vi "Executing.vi"(8 "error in (no error)":errorcluster, 11 "Command Actor in":refnum<class "Command Actor.lvclass">) -> (0 "error out":errorcluster, 3 "Command Actor out":refnum<class "Command Actor.lvclass">)   [LabVIEW 2013, in "Command Actor.lvlib" / "Command Actor.lvclass"]
uses:
  Command Actor.lvclass
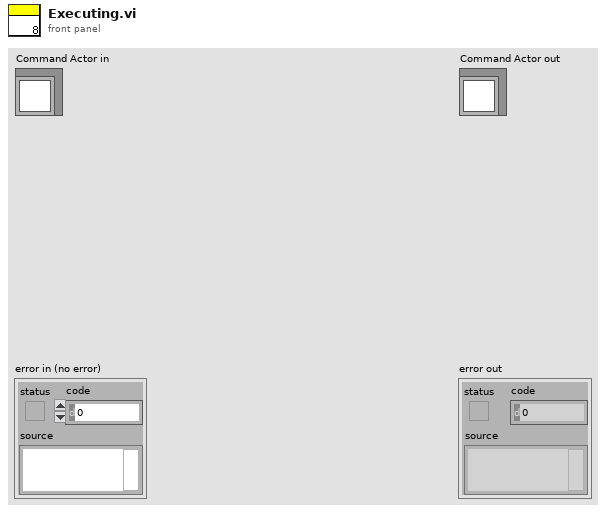
[diagram p1: front panel]
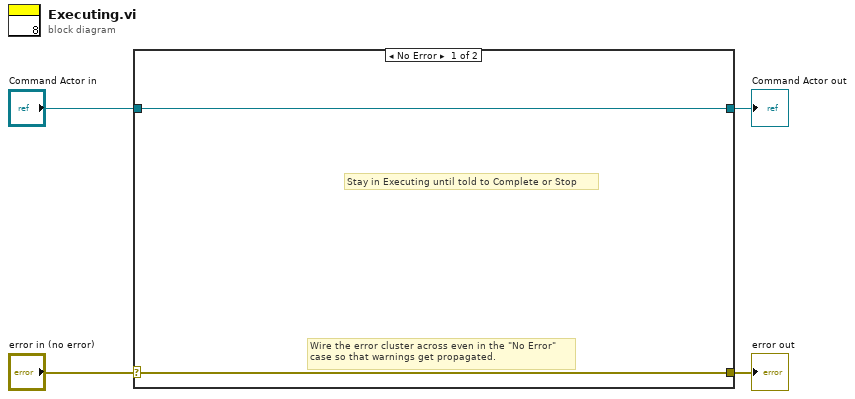
[diagram p0: block diagram]
diagram:
  n1 = case shown="No Error" "error in (no error)" {
    selector: "error in (no error)" -> [w6 w8]
    tunnel: [w6 w8] -> w3
    tunnel: [w5 w7] -> w1
    tunnel: "Command Actor in" -> [w5 w7]
    frame No Error {
      # "Stay in Executing until told to Complete or Stop"
      # "Wire the error cluster across even in the \"No Error\"\ncase so that warnings get propagated."
    }
    frame Error {
    }
  }
  "error out" <- w3
  "Command Actor out" <- w1
